vi "运维调试_总磷总氮.vi"() -> ()   [LabVIEW 2016, in "斯坦道总氮.lvlib"]
uses:
  <vilib>/Utility/miscctls.llb/LVPointTypeDef.ctl
  <vilib>/Plasmionique/MB Master/MB_Master/MB_Master.lvclass
  <vilib>/ptbypt/NI_PtbyPt.lvlib
panel:
  out "故障代码":u16
  out "告警代码":u16
  in  "产生故障":bool
  out "步骤":u16
  out "seconds since 1Jan1904 2":timestamp
  out "seconds since 1Jan1904":timestamp
  in  "周期设置":bool
  in  "流程操作":bool
  out "消解压力":sgl format="%#.2f kPa"
  out "权限等级":string
  out "总步数":i32
  out "滑动杆":dbl(slide) caption="测试进度" scale=0.0..100.0
  out "试剂余量显示":sgl[][](graph)
  in  "仪器校准":bool
  in  "参数查询":bool
  out "简易步骤名称":string
  in  "温度曲线":bool
  in  "试剂余量":bool
  in  "灯值调整":bool
  out "固件版本号":string
  out "模块版本号":string
  out "注射器温度":sgl format="%#.2f ℃"
  out "消解温度":sgl format="%#.2f ℃"
  out "ADC":sgl
  out "F3":sgl format="%#.6f"
  out "F2":sgl format="%#.6f"
  out "F1":sgl format="%#.6f"
  out "F0":sgl format="%#.6f"
  out "运行状态":T1 {"数据时间:" format="%<%y/%m/%d %H:%M:%S>T"; "仪器时间:" format="%<%y/%m/%d %H:%M:%S>T"}
  in  "单选按钮":T2=enum."总氮"
  in  "布尔":bool
  in  "外设固件":bool
  out "字符串 2":string
  in  "数组":string[](array[string])
  in  "返回":bool
  in  "参数设置":bool
  out "集成报警信息":string
  in  "停止":bool
  in  "手动启动":bool
  in  "调试":bool
  out "多列列表框":i32(listbox)
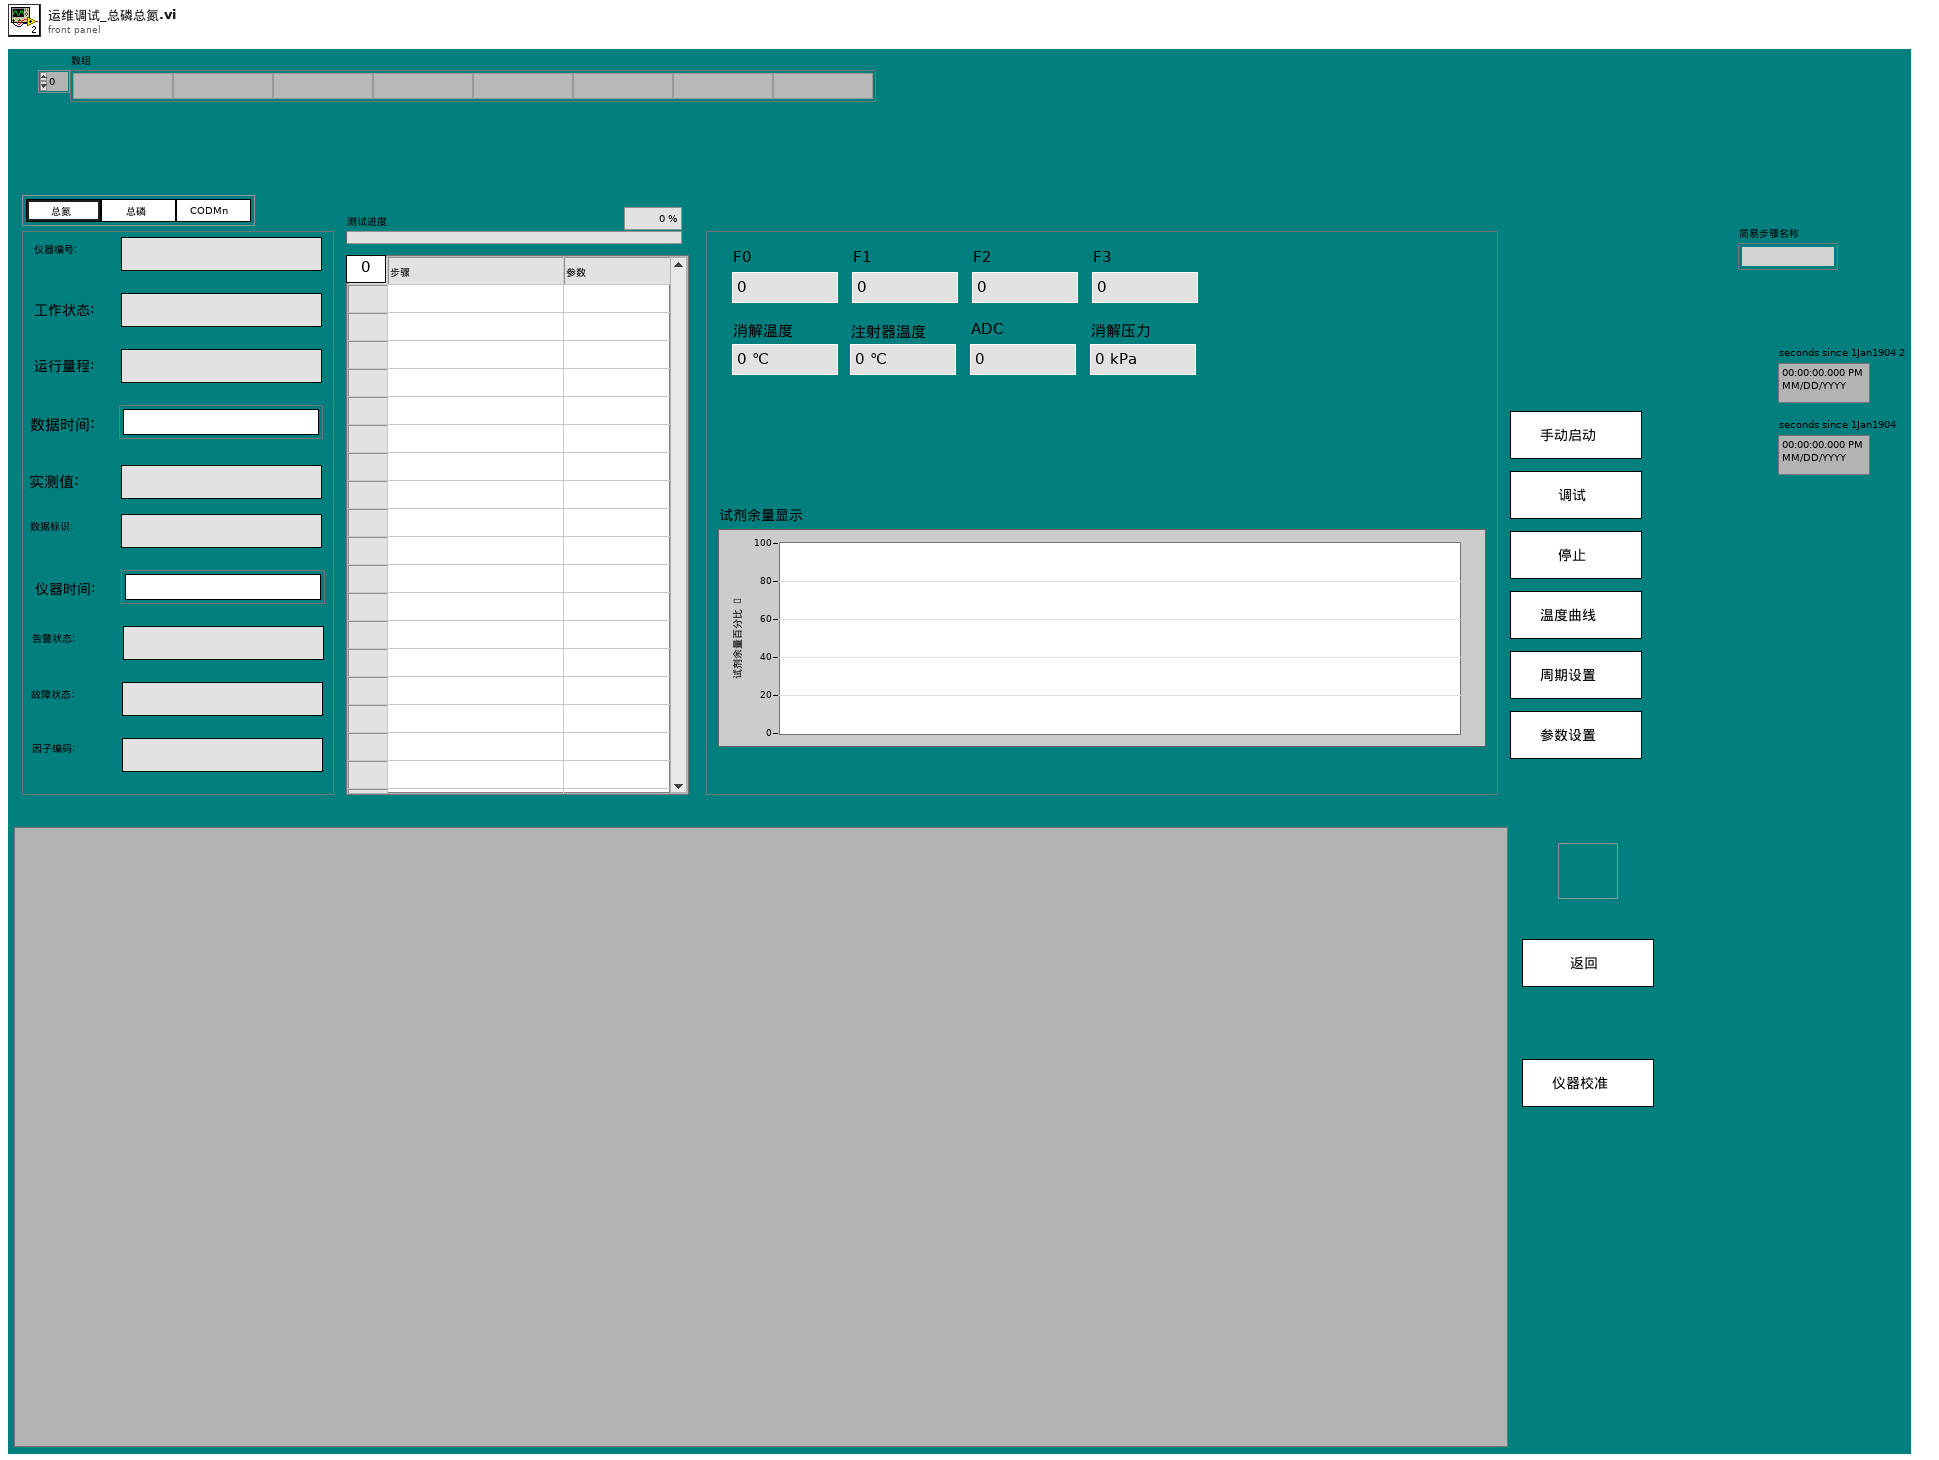
[diagram p1: front panel]
types:
  T1 = cluster{"仪器编号:":string, "工作状态:":string, "运行量程: ":string, "数据时间:":timestamp, "实测值:":string, "数据标识: ":string, "仪器时间:":timestamp, "告警状态: ":string, "故障状态:  ":string, "因子编码:":string}
  T2 = typedef "斯坦道总氮.lvlib/启动参数显示控件.ctl" = enum32{"COD", "氨氮", "总氮", "总磷", "磷酸盐", "硝氮", "亚硝氮", "硅酸盐", "硫化物", "氟化物", "CODMn"}
  T3 = typedef "报警信息字段定义.ctl" = cluster{"时间":timestamp, "参数":string, "元器件":string, "故障现象":string, "故障分析":string, "state":string, "code":string, "platform_alarm_code":string, "是否上报":string}
  T4 = cluster{"系统时间":timestamp, "工作状态":u16, "测量模式":enum16{"待机", "连续模式", "周期模式", "定点模式", "受控模式", "手动模式"}, "告警代码":u16, "故障代码":u16, "日志代码":u16, "软件版本":u16, "F0":sgl, "F1":sgl, "F2":sgl, "F3":sgl, "T":sgl, "H":sgl, "id":u16, "flowid":u16, "量程":u16, "总磷控温温度1":sgl, "营养盐控温温度2":sgl, "ADC":sgl, "结果值":sgl, "运行时间":u16, "步骤详情":string, "步骤流程":string}
  T5 = typedef "Alarm interface.lvlib/报警短信语音交互.ctl" = cluster{"参数":string, "元器件":string, "故障现象":string, "code":string, "platform_alarm_code":string, "solutionList":cluster{"reason":string, "solution":string}[], "是否上报":string}
  T6 = typedef "LVPointTypeDef.ctl" = cluster{"Horizontal":i16, "Vertical":i16}
  T7 = cluster{"Major":u16, "Minor":u16, "Fix":u16, "Build":u16}
  T8 = typedef "LVStringsAndValuesArrayTypeDef_U16.ctl" = cluster{"String":string, "Value":u16}[]
  T9 = cluster{"因子编码":u32, "单位":u16, "标样参考值":sgl, "水样数据时间":timestamp, "水样实测值":sgl, "水样数据标识":string, "标样数据时间":timestamp, "标样实测值":sgl, "标样数据标识":string, "空白数据时间":timestamp, "空白实测值":sgl, "空白数据标识":string, "零点核查数据时间":timestamp, "零点核查实测值":sgl, "零点核查数据标识":string, "跨度核查数据时间":timestamp, "跨度核查实测值":sgl, "跨度核查数据标识":string, "加标回收数据时间":timestamp, "加标回收实测值":sgl, "加标回收数据标识":string, "平行样数据时间":timestamp, "平行样实测值":sgl, "平行样数据标识":string, "F0":sgl, "F1":sgl, "F2":sgl, "F3":sgl, "F4":sgl, "F5":sgl, "F6":sgl, "F7":sgl, "温度":sgl, "湿度":sgl, "X值":sgl, "fidrange":u16, "X1值":sgl}[]
  T10 = typedef "SingleStepTestV3.lvlib/SingleStepTestV3.lvclass/仪器版本.ctl" = enum16{"V3.1版", "V4版", "V3版", "V4.2版"}
  T11 = cluster{"因子编码":u32, "单位":u16, "标样参考值":sgl, "水样数据时间":timestamp, "水样实测值":sgl, "水样数据标识":string, "标样数据时间":timestamp, "标样实测值":sgl, "标样数据标识":string, "空白数据时间":timestamp, "空白实测值":sgl, "空白数据标识":string, "零点核查数据时间":timestamp, "零点核查实测值":sgl, "零点核查数据标识":string, "跨度核查数据时间":timestamp, "跨度核查实测值":sgl, "跨度核查数据标识":string, "加标回收数据时间":timestamp, "加标回收实测值":sgl, "加标回收数据标识":string, "平行样数据时间":timestamp, "平行样实测值":sgl, "平行样数据标识":string, "F0":sgl, "F1":sgl, "F2":sgl, "F3":sgl, "F4":sgl, "F5":sgl, "F6":sgl, "F7":sgl, "温度":sgl, "湿度":sgl, "X值":sgl, "fidrange":u16, "X1值":sgl}
  T12 = typedef "TimingControl.lvlib/TimingControl.lvclass/国标控制命令.ctl" = enum16{"启动测量", "标样核查", "零点核查", "跨度核查", "空白测试", "平行样测试", "加标回收", "空白校准", "标样校准", "初始化（清洗）", "停止测试", "仪器重启", "校时", "模式设置", "测量间隔设置"}
  T13 = typedef "TimingControl.lvlib/TimingControl.lvclass/测量参数.ctl" = u16
  T14 = enum32{"Bad", "Idle", "Run top level", "Running"}
  T15 = cluster{"时间标识":timestamp, "设备":string, "日志信息":string, "流程参数":string}
  T16 = typedef "LVRowAndColumnUnsignedTypeDef.ctl" = cluster{"Row":u32, "Column":u32}
  T17 = typedef "操作日志字段定义.ctl" = cluster{"时间":timestamp, "参数":string, "日志信息":string, "流程参数":string}
  T18 = cluster{"站号":u16, "量程切换":enum32{"H", "L", "AUTO"}, "控制命令":enum16{"启动测量", "标样核查", "零点核查", "跨度核查", "空白测试", "平行样测试", "加标回收", "空白校准", "标样校准", "初始化（清洗）", "停止测试", "仪器重启", "校时", "模式设置", "测量间隔设置"}, "模式设置":enum16{"待机", "连续模式", "周期模式", "定点模式", "受控模式", "手动模式"}, "测量间隔":u16}
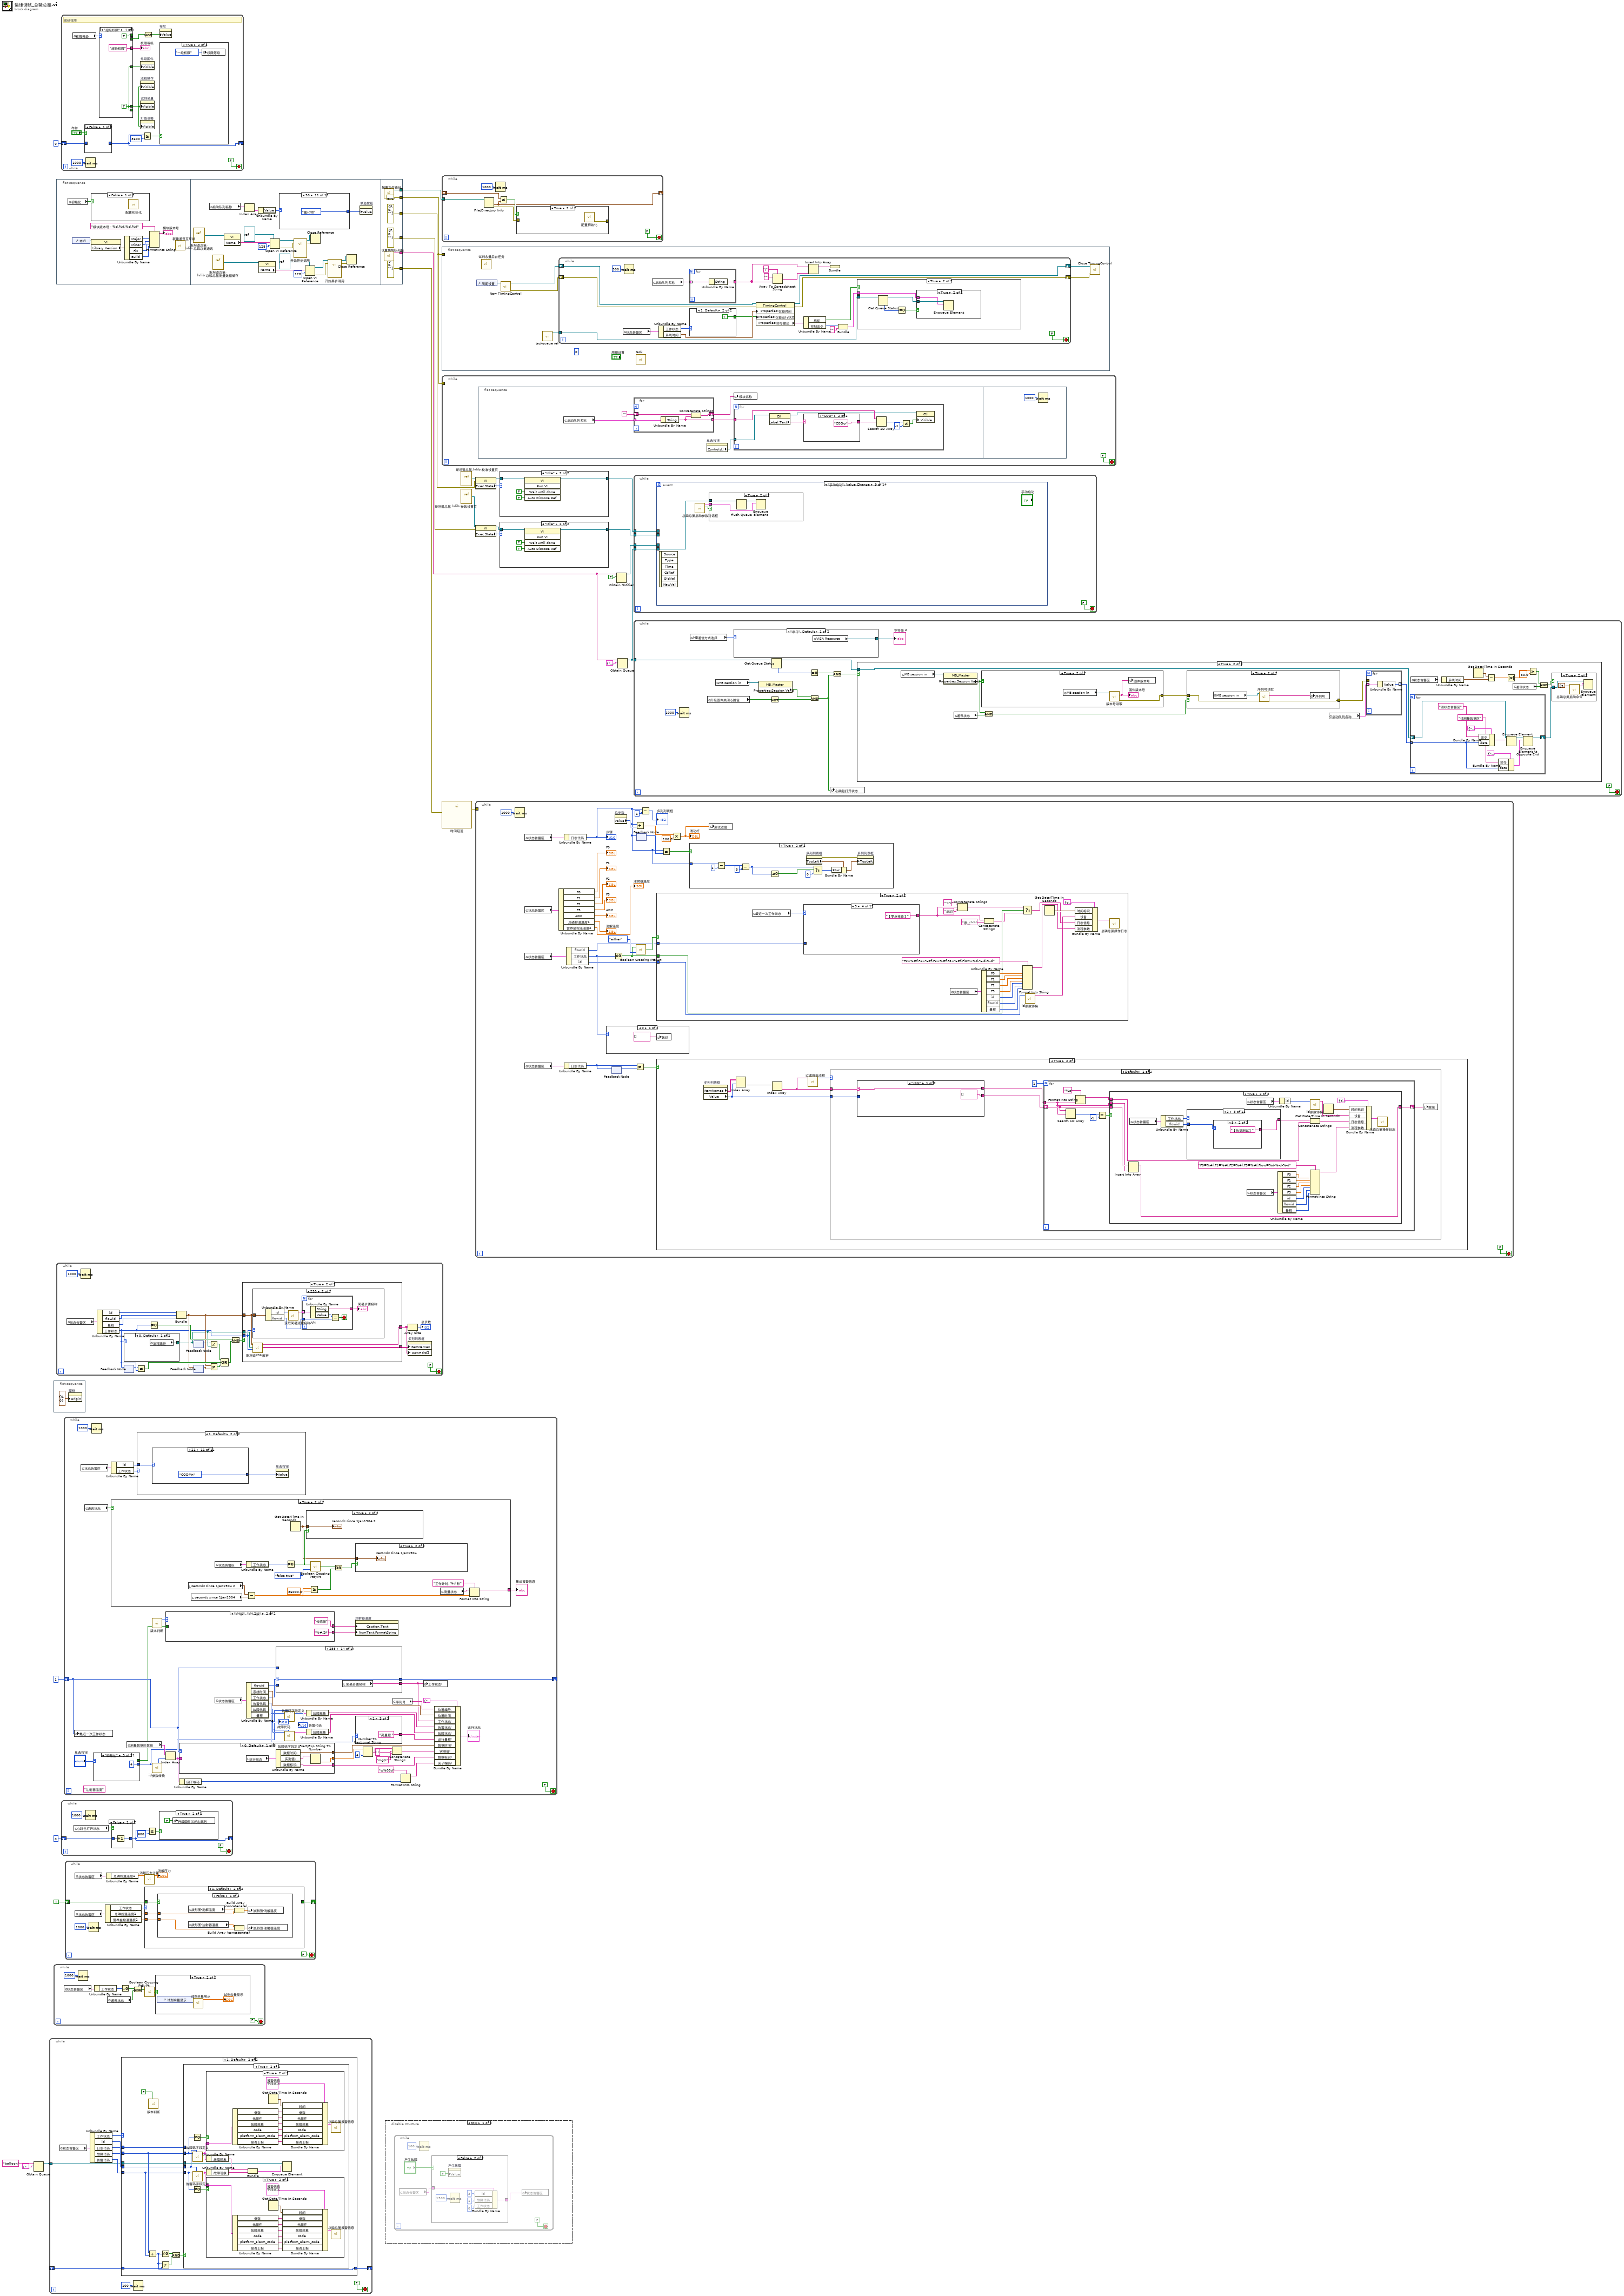
[diagram p0: block diagram]
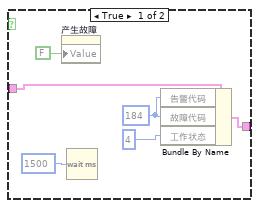
[diagram p2: hidden frame]
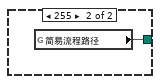
[diagram p8: hidden frame]
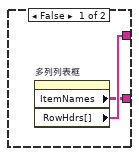
[diagram p9: hidden frame]
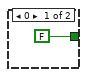
[diagram p13: hidden frame]
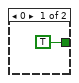
[diagram p20: hidden frame]
diagram:
  n1 = Obtain Queue(name (unnamed)="balloon" ("名称（未命名）"), element data type=cluster{"Title":string, "Body":string} {"Title"="", "Body"=""}) -> (queue out=w1:refnum<queue>)  [unwired: 3 in, 2 out]
  n2 = while {
    shift-right: [w29] -> _
    shift-left: _ -> [w31]
    tunnel: w1 -> [w28]
    stop <- FALSE stop-if-true
    n3 = global read "VAR总磷总氮全局变量.vi" "状态告警区"() -> (w27:T4)
    n4 = Unbundle By Name(w27) -> ("工作状态"=w36:u16, "id"=w35:u16, "日志代码"=w34:u16, "故障代码"=w33:u16, "告警代码"=w32:u16)
    n5 = case shown="1, Default" w36 {
      tunnel: w35 -> [_ w41]
      tunnel: w34 -> [_ w44]
      tunnel: w33 -> [_ w43]
      tunnel: w32 -> [_ w42]
      tunnel: w31 -> [w38 w47]
      tunnel: [w38 w45] -> w29
      tunnel: w28 -> [_ w40]
      frame 0 {
      }
      frame 1, Default {
        n6 = Add(x=w43, y=w42) -> (x+y=w45:u16)
        n7 = call "版本判断.vi"("Extern"=FALSE) -> ()  [unwired: 10 in, 1 out]
        n8 = Not Equal To 0?(x=w45) -> (x != 0?=w49:bool)
        n9 = Not Equal?(x=w45, y=w47) -> (x != y?=w48:bool)
        n10 = And(x=w49, y=w48) -> (x .and. y?=w46:bool)
        n11 = case shown="True" w46 {
          tunnel: w44 -> [_ _]
          tunnel: w43 -> [_ w54]
          tunnel: w42 -> [_ w51]
          tunnel: w41 -> [_ w50]
          tunnel: w40 -> [_ w58]
          frame False {
          }
          frame True {
            n12 = Not Equal To 0?(x=w54) -> (x != 0?=w56:bool)
            n13 = Not Equal To 0?(x=w51) -> (x != 0?=w55:bool)
            n14 = call "故障码字段定义.vi"("id"=w50, "故障代码"=w54) -> ("告警信息"=w53:T5)  [unwired: 9 in]
            n15 = call "告警码字段定义.vi"("id"=w50, "告警代码"=w51) -> ("告警信息"=w52:T5)  [unwired: 9 in]
            n16 = case shown="True" w56 {
              tunnel: w53 -> [_ w78]
              frame False {
              }
              frame True {
                n17 = Unbundle By Name(w78) -> ("参数"=w77:string, "元器件"=w76:string, "故障现象"=w75:string, "code"=w74:string, "platform_alarm_code"=w73:string, "是否上报"=w72:string)
                n18 = Get Date/Time In Seconds() -> (seconds since 1Jan1904=w79:timestamp)
                n19 = Bundle By Name(cluster=T3 {"时间"=timestamp(0 s since 1904-01-01), "参数"="", "元器件"="", "故障现象"="", "故障分析"="", "state"="", "code"="", "platform_alarm_code"="", "是否上报"=""} ("data in"), "时间"=w79, "参数"=w77, "元器件"=w76, "故障现象"=w75, "code"=w74, "platform_alarm_code"=w73, "是否上报"=w72) -> (w71:T3)
                n20 = call "总磷总氮报警信息.vi"("data in"=w71) -> ()  [unwired: 10 in, 1 out]
              }
            }
            n21 = Unbundle By Name(w53) -> ("故障现象"=w60:string)
            n22 = Unbundle By Name(w52) -> ("故障现象"=w59:string)
            n23 = case shown="True" w55 {
              tunnel: w52 -> [_ w62]
              frame False {
              }
              frame True {
                n24 = Unbundle By Name(w62) -> ("参数"=w65:string, "元器件"=w66:string, "故障现象"=w67:string, "code"=w68:string, "platform_alarm_code"=w69:string, "是否上报"=w70:string)
                n25 = Get Date/Time In Seconds() -> (seconds since 1Jan1904=w64:timestamp)
                n26 = Bundle By Name(cluster=T3 {"时间"=timestamp(0 s since 1904-01-01), "参数"="", "元器件"="", "故障现象"="", "故障分析"="", "state"="", "code"="", "platform_alarm_code"="", "是否上报"=""} ("data in"), "时间"=w64, "参数"=w65, "元器件"=w66, "故障现象"=w67, "code"=w68, "platform_alarm_code"=w69, "是否上报"=w70) -> (w61:T3)
                n27 = call "总磷总氮报警信息.vi"("data in"=w61) -> ()  [unwired: 10 in, 1 out]
              }
            }
            n28 = Bundle("故障现象"=w60, "故障现象"=w59) -> (w57:cluster{"故障现象":string, "故障现象":string})  [unwired: 1 in]
            n29 = Enqueue Element(queue=w58, element=w57) -> ()  [unwired: 2 in, 3 out]
          }
        }
      }
    }
    n30 = Wait (ms)(milliseconds to wait=u32 100 ("等待时间（毫秒）")) -> ()  [unwired: 1 out]
  }
  n31 = flat-sequence {
    frame #0 {
      n32 = property on="窗格" class="Pane"("Origin"=T6 {"Horizontal"=0, "Vertical"=0} ("原点")) -> ()  [unwired: 2 in, 2 out]
    }
  }
  n33 = while {
    stop <- FALSE stop-if-true
    n34 = global read "VAR总磷总氮全局变量.vi" "状态告警区"() -> (w86:T4)
    n35 = Wait (ms)(milliseconds to wait=u32 1000 ("等待时间（毫秒）")) -> ()  [unwired: 1 out]
    n36 = Unbundle By Name(w86) -> ("工作状态"=w84:u16)
    n37 = global read "VAR总磷总氮全局变量.vi" "通讯状态"() -> (w87:bool)
    n38 = Equal To 0?(x=w84) -> (x = 0?=w83:bool)
    n39 = And(x=w83, y=w87) -> (x .and. y?=w85:bool)
    n40 = call <vilib>:"Boolean Crossing PtByPt.vi"("input"=w85) -> ("crossing"=w82:bool)  [unwired: 2 in]
    n41 = case shown="True" w82 {
      frame False {
      }
      frame True {
        n42 = control-ref of="试剂余量显示"() -> (w90:refnum<vi>)
        n43 = call "试剂余量展示.vi"("波形图 2"=w90) -> ("波形图"=→"试剂余量显示":sgl[][])  [unwired: 10 in]
      }
    }
  }
  n44 = flat-sequence {
    tunnel: [w138] -> w20
    tunnel: [errorcluster {"status"=FALSE, "code"=0, "source"=""} ("错误输入（无错误）")] -> w11
    tunnel: [errorcluster {"status"=FALSE, "code"=0, "source"=""} ("错误输入（无错误）")] -> w10
    tunnel: [w135] -> w8
    tunnel: [errorcluster {"status"=FALSE, "code"=0, "source"=""} ("error out")] -> w7
    tunnel: [errorcluster {"status"=FALSE, "code"=0, "source"=""} ("错误输入（无错误）")] -> w6
    frame #0 {
      n45 = global read "VAR总磷总氮全局变量.vi" "初始化"() -> (w92:bool)
      n46 = control-ref of="本VI"() -> (w100:refnum<vi>)
      n47 = case shown="False" w92 {
        frame False {
          n48 = call "配置初始化.vi"() -> ()  [unwired: 11 in, 1 out]
        }
        frame True {
        }
      }
      n49 = property class="VI"(reference=w100) -> ("Library.Version"=w99:T7)  [unwired: 1 in, 2 out]
      n50 = Unbundle By Name(w99) -> ("Major"=w97:u16, "Minor"=w96:u16, "Fix"=w95:u16, "Build"=w94:u16)
      n51 = Format Into String(format string="模块版本号：%d.%d.%d.%d" ("格式字符串"), w97, w96, w95, w94) -> (resulting string=→"模块版本号":string)  [unwired: 2 in, 1 out]
      n52 = call "新建通讯互斥锁.vi"() -> ()  [unwired: 11 in, 1 out]
    }
    frame #1 {
      n53 = vi-ref "斯坦道总氮.lvlib:总磷总氮通讯.vi"() -> (w105:refnum<vi>)
      n54 = global read "model config var.vi" "启动队列名称"() -> (w103:cluster{"String":string, "Value":u16}[])
      n55 = vi-ref "斯坦道总氮.lvlib:总磷总氮测量数据储存.vi"() -> (w113:refnum<vi>)
      n56 = property class="VI"(reference=w105) -> ("Name"=w106:string)  [unwired: 1 in, 2 out]
      n57 = Index Array(array=w103) -> (element=w102:cluster{"String":string, "Value":u16})  [unwired: 1 in]
      n58 = Unbundle By Name(w102) -> ("Value"=w101:u16)
      n59 = property class="VI"(reference=w113) -> ("Name"=w120:string)  [unwired: 1 in, 2 out]
      n60 = Open VI Reference(type specifier VI Refnum (for type only)=refnum<vi> refnum, vi path=w106, options=128 ("选项")) -> (vi reference=w108:refnum<vi>, error out=w110:errorcluster)  [unwired: 3 in]
      n61 = case shown="50" w101 {
        tunnel: [w121 启动参数显示控件."总磷" ("单选按钮") 启动参数显示控件."总氮" ("单选按钮") 启动参数显示控件."COD" ("单选按钮") 启动参数显示控件."氨氮" ("单选按钮") 启动参数显示控件."磷酸盐" ("单选按钮") 启动参数显示控件."硝氮" ("单选按钮") 启动参数显示控件."亚硝氮" ("单选按钮") 启动参数显示控件."硅酸盐" ("单选按钮") 启动参数显示控件."硫化物" ("单选按钮") 启动参数显示控件."氟化物" ("单选按钮") 启动参数显示控件."CODMn" ("单选按钮")] -> w104
        frame 0, Default {
          n62 = property on="单选按钮" class="RadioBtnsControl (strict)"() -> ("Value"=w121:T2)  [unwired: 2 in, 2 out]
        }
        frame 1 {
        }
        frame 2 {
        }
        frame 22 {
        }
        frame 3 {
        }
        frame 4 {
        }
        frame 5 {
        }
        frame 6 {
        }
        frame 7 {
        }
        frame 8 {
        }
        frame 50 {
        }
        frame 21 {
        }
      }
      n63 = call-by-ref "开始异步调用"(reference=w108, error in=w110) -> (reference out=w112:refnum<vi>, error out=w111:errorcluster)  [unwired: 12 in]
      n64 = Open VI Reference(type specifier VI Refnum (for type only)=refnum<vi> refnum, vi path=w120, options=128 ("选项")) -> (vi reference=w118:refnum<vi>, error out=w116:errorcluster)  [unwired: 3 in]
      n65 = Close Reference(reference=w112, error in (no error)=w111) -> ()  [unwired: 1 out]
      n66 = call-by-ref "开始异步调用"(reference=w118, error in=w116) -> (reference out=w114:refnum<vi>, error out=w115:errorcluster)  [unwired: 12 in]
      n67 = Close Reference(reference=w114, error in (no error)=w115) -> ()  [unwired: 1 out]
      n68 = property on="单选按钮" class="RadioBtnsControl (strict)"("Value"=w104) -> ()  [unwired: 2 in, 2 out]
    }
    frame #2 {
      n69 = call "配置文件路径.vi"() -> ("appended path"=w135:path)  [unwired: 11 in]
      n70 = call "设置模块队列名.vi"() -> ("Msg"=w138:string)  [unwired: 5 in]
    }
  }
  n71 = while {
    stop <- FALSE stop-if-true
    n72 = global read "VAR总磷总氮全局变量.vi" "状态告警区"() -> (w150:T4)
    n73 = Wait (ms)(milliseconds to wait=u32 1000 ("等待时间（毫秒）")) -> ()  [unwired: 1 out]
    n74 = Unbundle By Name(w150) -> ("id"=w149:u16, "flowid"=w148:u16, "量程"=w147:u16, "工作状态"=w140:u16)
    n75 = case shown="0, Default" w140 {
      tunnel: [w160 w161] -> w142
      frame 0, Default {
        n76 = global read "总磷总氮断电保存全局变量.vi" "流程路径"() -> (w160:path)
      }
      frame 255 {
        n77 = global read "总磷总氮断电保存全局变量.vi" "简易流程路径"() -> (w161:path)
      }
    }
    n78 = feedback #1() -> (w139:u16)  [unwired: 1 in]
    n79 = feedback-in #1(w140) -> ()
    n80 = Not Equal?(x=w139, y=w140) -> (x != y?=w156:bool)
    n81 = Not Equal To 0?(x=w140) -> (x != 0?=w151:bool)
    n82 = Bundle("id"=w149, "flowid"=w148, "量程"=w147) -> (w144:cluster{"id":u16, "flowid":u16, "量程":u16})  [unwired: 1 in]
    n83 = feedback #2() -> (w141:path)  [unwired: 1 in]
    n84 = feedback-in #2(w142) -> ()
    n85 = feedback-in #3(w144) -> ()
    n86 = feedback #3() -> (w145:cluster{"id":u16, "flowid":u16, "量程":u16})  [unwired: 1 in]
    n87 = Not Equal?(x=w141, y=w142) -> (x != y?=w155:bool)
    n88 = Not Equal?(x=w144, y=w145) -> (x != y?=w143:bool)
    n89 = Compound Arithmetic op=OR ("复合运算")(w155, w156, w143) -> (w157:bool)
    n90 = And(x=w151, y=w157) -> (x .and. y?=w152:bool)
    n91 = case shown="True" w152 {
      tunnel: [w163 w166] -> w154
      tunnel: [w162 w167] -> w158
      tunnel: w144 -> [_ w165]
      tunnel: w142 -> [_ w168]
      tunnel: w140 -> [_ w164]
      frame False {
        n92 = property on="多列列表框" class="MCListbox (strict)"() -> ("ItemNames"=w162:string[][], "RowHdrs[]"=w163:string[])  [unwired: 2 in, 2 out]
      }
      frame True {
        n93 = case shown="255" w164 {
          tunnel: w165 -> [_ w173]
          frame 0, Default {
          }
          frame 255 {
            n94 = Unbundle By Name(w173) -> ("id"=w172:u16, "flowid"=w170:u16)
            n95 = call "获取简易流程名称API.vi"("参数下拉列表"=w172) -> ("字符串与值[]"=w171:T8)  [unwired: 9 in, 1 out]
            n96 = for {
              tunnel: w171 -> [w178] mode=indexing
              tunnel: w170 -> [w176]
              tunnel: [w175] -> w169
              stop <- w174 stop-if-true
              n97 = Unbundle By Name(w178) -> ("String"=w175:string, "Value"=w177:u16)
              n98 = Equal?(x=w177, y=w176) -> (x = y?=w174:bool)
            }
            "简易步骤名称" <- w169
          }
        }
        n99 = call "斯坦道XML解析.vi"("工作状态"=w164, "添加的路径"=w168, "参数簇"=w165) -> ("步骤名"=w167:string[][], "索引"=w166:string[])  [unwired: 6 in, 1 out]
      }
    }
    n100 = Array Size(array=w154) -> (size(s)=→"总步数":i32)
    n101 = property on="多列列表框" class="MCListbox (strict)"("ItemNames"=w158, "RowHdrs[]"=w154) -> ()  [unwired: 2 in, 2 out]
  }
  n102 = while {
    shift-right: [w188] -> _
    shift-left: u32 0 ("y") -> [w190]
    stop <- FALSE stop-if-true
    # "密码权限"
    n103 = global read "VAR总磷总氮全局变量.vi" "权限等级"() -> (w185:enum16{"一级权限", "二级权限", "三级权限", "超级权限"})
    n104 = case shown="False" "布尔" {
      tunnel: w190 -> [_ w203]
      tunnel: [_ w202] -> w188
      frame False {
      }
      frame True {
        n105 = Increment(x=w203) -> (x+1=w202:u32)
      }
    }
    n106 = Wait (ms)(milliseconds to wait=u32 1000 ("等待时间（毫秒）")) -> ()  [unwired: 1 out]
    n107 = case shown="\"超级权限\"" w185 {
      tunnel: [_ w195 w197 w200] -> w179
      tunnel: [_ _ w197 w200] -> _
      tunnel: [_ w195 w197 w200] -> w184
      tunnel: [_ _ _ TRUE] -> _
      tunnel: [TRUE _ _ _] -> w182
      tunnel: ["一级权限" "二级权限" "三级权限" "超级权限"] -> w180
      frame "一级权限", Default {
      }
      frame "二级权限" {
        w195 = TRUE
      }
      frame "三级权限" {
        w197 = TRUE
      }
      frame "超级权限" {
        w200 = TRUE
      }
    }
    "权限等级" <- w180
    n108 = property on="外设固件" class="Bool"("Visible"=w184) -> ()  [unwired: 2 in, 2 out]
    n109 = property on="流程操作" class="Bool"("Visible"=w179) -> ()  [unwired: 2 in, 2 out]
    n110 = property on="试剂余量" class="Bool"("Visible"=w179) -> ()  [unwired: 2 in, 2 out]
    n111 = property on="灯值调整" class="Bool"("Visible"=w179) -> ()  [unwired: 2 in, 2 out]
    n112 = Greater Or Equal?(x=w188, y=u32 3600) -> (x >= y?=w186:bool)
    n113 = Not(x=w182) -> (.not. x?=w181:bool)
    n114 = property on="布尔" class="Bool (strict)"("Value"=w181) -> ()  [unwired: 2 in, 2 out]
    n115 = case shown="True" w186 {
      frame False {
      }
      frame True {
        n116 = global write "VAR总磷总氮全局变量.vi" "权限等级"(enum16{"一级权限", "二级权限", "三级权限", "超级权限"}."一级权限" ("权限等级")) -> ()
      }
    }
  }
  n117 = while {
    shift-right: [w208] -> _
    shift-left: 0 -> [w209]
    stop <- FALSE stop-if-true
    n118 = global read "VAR总磷总氮全局变量.vi" "心跳包打开状态"() -> (w204:bool)
    n119 = Wait (ms)(milliseconds to wait=u32 1000 ("等待时间（毫秒）")) -> ()  [unwired: 1 out]
    n120 = case shown="False" w204 {
      tunnel: w209 -> [w213 _]
      tunnel: [w212 _] -> w208
      frame False {
        n121 = Increment(x=w213) -> (x+1=w212:i32)
      }
      frame True {
      }
    }
    n122 = Greater Or Equal?(x=w208, y=600) -> (x >= y?=w206:bool)
    n123 = case shown="True" w206 {
      frame False {
      }
      frame True {
        n124 = global write "VAR总磷总氮全局变量.vi" "升级固件关闭心跳包"(FALSE ("关闭心跳包")) -> ()
      }
    }
  }
  n125 = while {
    shift-right: [w225] -> _
    shift-left: u16 1 ("工作状态") -> [w223]
    stop <- FALSE stop-if-true
    (unwired) "注射器温度"
    n126 = global write "VAR总磷总氮全局变量.vi" "最近一次工作状态"(w223) -> ()
    n127 = global read "VAR总磷总氮全局变量.vi" "状态告警区"() -> (w245:T4)
    n128 = global read "VAR总磷总氮全局变量.vi" "通讯状态"() -> (w256:bool)
    n129 = Wait (ms)(milliseconds to wait=u32 1000 ("等待时间（毫秒）")) -> ()  [unwired: 1 out]
    n130 = case shown="\"磷酸盐\"" "单选按钮" {
      tunnel: [22 3 2 1 4 5 6 7 8 50 21] -> w214
      tunnel: [_ TRUE _ _ _ _ _ _ _ _ _] -> w217
      frame "COD", Default {
      }
      frame "氨氮" {
      }
      frame "总氮" {
      }
      frame "总磷" {
      }
      frame "磷酸盐" {
      }
      frame "硝氮" {
      }
      frame "亚硝氮" {
      }
      frame "硅酸盐" {
      }
      frame "硫化物" {
      }
      frame "氟化物" {
      }
      frame "CODMn" {
      }
    }
    n131 = Unbundle By Name(w245) -> ("id"=w244:u16, "工作状态"=w240:u16)
    n132 = case shown="True" w256 {
      tunnel: ["通讯异常" ("集成报警信息") w375] -> w255
      frame False {
      }
      frame True {
        n133 = local read "seconds since 1Jan1904 2"() -> (w367:timestamp)
        n134 = local read "seconds since 1Jan1904"() -> (w370:timestamp)
        n135 = global read "VAR总磷总氮全局变量.vi" "状态告警区"() -> (w377:T4)
        n136 = Unbundle By Name(w377) -> ("工作状态"=w373:u16)
        n137 = Subtract(x=w367, y=w370) -> (x-y=w366:dbl)
        n138 = Not Equal To 0?(x=w373) -> (x != 0?=w369:bool)
        n139 = Get Date/Time In Seconds() -> (seconds since 1Jan1904=w368:timestamp)
        n140 = case shown="True" w369 {
          tunnel: w368 -> [_ w378]
          frame False {
          }
          frame True {
            "seconds since 1Jan1904 2" <- w378
          }
        }
        n141 = Greater Or Equal?(x=w366, y=36000.0) -> (x >= y?=w363:bool)
        n142 = call <vilib>:"Boolean Crossing PtByPt.vi"("direction"=enum16{"either", "false-true", "true-false"}."false-true", "input"=w369) -> ("crossing"=w371:bool)  [unwired: 1 in]
        n143 = Or(x=w371, y=w363) -> (x .or. y?=w364:bool)
        n144 = case shown="True" w364 {
          tunnel: w368 -> [_ w379]
          frame False {
          }
          frame True {
            "seconds since 1Jan1904" <- w379
          }
        }
        n145 = global read "VAR总磷总氮全局变量.vi" "测量状态"() -> (w374:string)
        n146 = Format Into String(format string="工作计时: %d 秒" ("格式字符串"), initial string=w374, w366) -> (resulting string=w375:string)  [unwired: 1 in, 1 out]
      }
    }
    "集成报警信息" <- w255
    n147 = global read "VAR总磷总氮全局变量.vi" "测量数据区数组"() -> (w229:T9)
    n148 = case shown="1, Default" w240 {
      tunnel: w244 -> [_ w312]
      frame 0 {
      }
      frame 1, Default {
        n149 = case shown="21" w312 {
          tunnel: [w313 启动参数显示控件."总磷" ("单选按钮") 启动参数显示控件."总氮" ("单选按钮") 启动参数显示控件."COD" ("单选按钮") 启动参数显示控件."氨氮" ("单选按钮") 启动参数显示控件."磷酸盐" ("单选按钮") 启动参数显示控件."硝氮" ("单选按钮") 启动参数显示控件."亚硝氮" ("单选按钮") 启动参数显示控件."硅酸盐" ("单选按钮") 启动参数显示控件."硫化物" ("单选按钮") 启动参数显示控件."CODMn" ("单选按钮") 启动参数显示控件."氟化物" ("单选按钮")] -> w311
          frame 0, Default {
            n150 = property on="单选按钮" class="RadioBtnsControl (strict)"() -> ("Value"=w313:T2)  [unwired: 2 in, 2 out]
          }
          frame 1 {
          }
          frame 2 {
          }
          frame 22 {
          }
          frame 3 {
          }
          frame 4 {
          }
          frame 5 {
          }
          frame 6 {
          }
          frame 7 {
          }
          frame 8 {
          }
          frame 21 {
          }
          frame 50 {
          }
        }
        n151 = property on="单选按钮" class="RadioBtnsControl (strict)"("Value"=w311) -> ()  [unwired: 2 in, 2 out]
      }
    }
    n152 = call "版本判断.vi"() -> ("仪器版本"=w219:T10)  [unwired: 11 in]
    n153 = call "id参数转换.vi"("id"=w214) -> ("数组资源索引"=w226:i32)  [unwired: 9 in, 1 out]
    n154 = case shown="\"V4版\", \"V4.2版\"" w219 {
      tunnel: [w259 "传感器" ("标题.文本")] -> w216
      tunnel: ["%#.2f ℃" ("数值文本.格式字符串") "%#.2f " ("数值文本.格式字符串")] -> w218
      tunnel: w217 -> [w262 _]
      frame "V3.1版", Default {
        n155 = Select(t="显色温度", s=w262, f="注射器温度" ("标题.文本")) -> (s? t:f=w259:string)
      }
      frame "V4版", "V4.2版" {
      }
    }
    n156 = Index Array(array=w229, index=w226) -> (element=w228:T11)
    n157 = case shown="0, Default" w223 {
      tunnel: [w280 w286 w290 w294 w298 w302 w306 w310] -> w239
      tunnel: [w278 w285 w289 w293 w296 w301 w305 w309] -> w234
      tunnel: [w281 w284 w288 w292 w295 w300 w304 w308] -> w232
      tunnel: w228 -> [_ w283 w287 w291 w297 w299 w303 w307]
      frame 0, Default {
        n158 = local read "运行状态"() -> (w282:T1)
        n159 = Unbundle By Name(w282) -> ("数据时间:"=w280:timestamp, "实测值:"=w279:string, "数据标识:"=w281:string)
        n160 = Fract/Exp String To Number(string=w279) -> (number=w278:dbl)  [unwired: 3 in, 1 out]
      }
      frame 1 {
        n161 = Unbundle By Name(w283) -> ("水样数据时间"=w286:timestamp, "水样实测值"=w285:sgl, "水样数据标识"=w284:string)
      }
      frame 2, 9 {
        n162 = Unbundle By Name(w287) -> ("标样数据时间"=w290:timestamp, "标样实测值"=w289:sgl, "标样数据标识"=w288:string)
      }
      frame 3 {
        n163 = Unbundle By Name(w291) -> ("零点核查数据时间"=w294:timestamp, "零点核查实测值"=w293:sgl, "零点核查数据标识"=w292:string)
      }
      frame 4 {
        n164 = Unbundle By Name(w297) -> ("跨度核查数据时间"=w298:timestamp, "跨度核查实测值"=w296:sgl, "跨度核查数据标识"=w295:string)
      }
      frame 7 {
        n165 = Unbundle By Name(w299) -> ("加标回收数据时间"=w302:timestamp, "加标回收实测值"=w301:sgl, "加标回收数据标识"=w300:string)
      }
      frame 5, 8 {
        n166 = Unbundle By Name(w303) -> ("空白数据时间"=w306:timestamp, "空白实测值"=w305:sgl, "空白数据标识"=w304:string)
      }
      frame 6 {
        n167 = Unbundle By Name(w307) -> ("平行样数据时间"=w310:timestamp, "平行样实测值"=w309:sgl, "平行样数据标识"=w308:string)
      }
    }
    n168 = Unbundle By Name(w228) -> ("因子编码"=w230:u32)
    n169 = global read "VAR总磷总氮全局变量.vi" "状态告警区"() -> (w254:T4)
    n170 = Unbundle By Name(w254) -> ("flowid"=w222:u16, "系统时间"=w250:timestamp, "工作状态"=w249:u16, "告警代码"=w243:u16, "故障代码"=w242:u16, "量程"=w248:u16)
    "告警代码" <- w243
    "故障代码" <- w242
    n171 = case shown="255" w249 {
      selector: w249 -> [w329 _ w335 w339 w342 w344 w346 w348 w350 w352 w354 w356 w358 w361]
      tunnel: [w330 "空闲" ("工作状态") "水样测量" ("工作状态") w338 "零点核查" ("工作状态") "跨度核查" ("工作状态") "空白测试" ("工作状态") "平行样测试" ("工作状态") "加标回收" ("工作状态") "空白校准" ("工作状态") "标样校准" ("工作状态") "初始化" ("工作状态") "单步调试" ("工作状态") w360] -> w224
      tunnel: [w328 w333 w335 w339 w342 w344 w346 w348 w350 w352 w354 w356 w358 w361] -> w225
      tunnel: w223 -> [w328 w333 _ _ _ _ _ _ _ _ _ _ _ _]
      tunnel: w222 -> [_ _ _ w337 _ _ _ _ _ _ _ _ _ _]
      frame Default {
        n172 = Format Into String(format string="%d" ("格式字符串"), initial string="未知" ("工作状态"), w329) -> (resulting string=w330:string)  [unwired: 1 in, 1 out]
      }
      frame 0 {
      }
      frame 1 {
      }
      frame 2 {
        n173 = case shown="5" w337 {
          tunnel: ["标样核查" ("工作状态") "快捷测试" ("工作状态")] -> w338
          frame 0, Default {
          }
          frame 5 {
          }
        }
      }
      frame 3 {
      }
      frame 4 {
      }
      frame 5 {
      }
      frame 6 {
      }
      frame 7 {
      }
      frame 8 {
      }
      frame 9 {
      }
      frame 10 {
      }
      frame 254 {
      }
      frame 255 {
        n174 = local read "简易步骤名称"() -> (w360:string)
      }
    }
    n175 = call "告警码字段定义.vi"("id"=w214, "告警代码"=w243) -> ("告警信息"=w221:T5)  [unwired: 9 in]
    n176 = call "故障码字段定义.vi"("id"=w214, "故障代码"=w242) -> ("告警信息"=w241:T5)  [unwired: 9 in]
    n177 = Unbundle By Name(w221) -> ("故障现象"=w220:string)
    n178 = Unbundle By Name(w241) -> ("故障现象"=w215:string)
    n179 = property on="注射器温度" class="DigNum (strict)"("Caption.Text"=w216, "NumText.FormatString"=w218) -> ()  [unwired: 2 in, 2 out]
    n180 = case shown="1" w248 {
      tunnel: ["" ("字符串") "低量程 " ("字符串") "高量程 " ("字符串")] -> w247
      frame Default {
      }
      frame 0 {
      }
      frame 1 {
      }
    }
    n181 = Number To Fractional String(number=w234, precision (6)=i16 4 ("精度(6)")) -> (F-format string=w236:string)  [unwired: 2 in]
    n182 = Concatenate Strings(w236, " " ("字符串"), "mg/L" ("字符串")) -> (w233:string)
    n183 = global read "VAR总磷总氮全局变量.vi" "序列号"() -> (w251:string)
    n184 = Format Into String(format string="w%05d" ("格式字符串"), w230) -> (resulting string=w246:string)  [unwired: 2 in, 1 out]
    n185 = global write "VAR总磷总氮全局变量.vi" "工作状态:"(w224) -> ()
    n186 = Bundle By Name(cluster=T1 {"仪器编号:"="", "工作状态:"="", "运行量程: "="", "数据时间:"=timestamp(0 s since 1904-01-01), "实测值:"="", "数据标识: "="", "仪器时间:"=timestamp(0 s since 1904-01-01), "告警状态: "="", "故障状态:  "="", "因子编码:"=""} ("运行状态"), "仪器编号:"=w251, "仪器时间:"=w250, "工作状态:"=w224, "告警状态:"=w220, "故障状态:"=w215, "运行量程:"=w247, "数据时间:"=w239, "实测值:"=w233, "数据标识:"=w232, "因子编码:"=w246) -> (→"运行状态":T1)
  }
  n187 = while {
    shift-right: [w381] -> _
    shift-left: TRUE -> [w382]
    stop <- FALSE stop-if-true
    n188 = global read "VAR总磷总氮全局变量.vi" "状态告警区"() -> (w385:T4)
    n189 = global read "VAR总磷总氮全局变量.vi" "状态告警区"() -> (w388:T4)
    n190 = Wait (ms)(milliseconds to wait=u32 1000 ("等待时间（毫秒）")) -> ()  [unwired: 1 out]
    n191 = Unbundle By Name(w388) -> ("工作状态"=w383:u16, "总磷控温温度1"=w387:sgl, "营养盐控温温度2"=w386:sgl)
    n192 = Unbundle By Name(w385) -> ("总磷控温温度1"=w384:sgl)
    n193 = call "消解压力计算.vi"("当前消解温度"=w384) -> ("消解压力"=→"消解压力":dbl)  [unwired: 10 in]
    n194 = case shown="1, Default" w383 {
      tunnel: w387 -> [_ w394]
      tunnel: w386 -> [_ w393]
      tunnel: w382 -> [_ w392]
      tunnel: [TRUE _] -> w381
      frame 0 {
      }
      frame 1, Default {
        n195 = case shown="False" w392 {
          tunnel: w394 -> [w400 _]
          tunnel: w393 -> [w399 _]
          frame False {
            n196 = global read "VAR总磷总氮全局变量.vi" "波形图-消解温度"() -> (w398:sgl[])
            n197 = global read "VAR总磷总氮全局变量.vi" "波形图-注射器温度"() -> (w397:sgl[])
            n198 = Build Array (concatenate)(w398, w400) -> (w396:sgl[])
            n199 = Build Array (concatenate)(w397, w399) -> (w395:sgl[])
            n200 = global write "VAR总磷总氮全局变量.vi" "波形图-消解温度"(w396) -> ()
            n201 = global write "VAR总磷总氮全局变量.vi" "波形图-注射器温度"(w395) -> ()
          }
          frame True {
            w401 = dbl[] [] ("波形图-消解温度")
            n202 = global write "VAR总磷总氮全局变量.vi" "波形图-消解温度"(w401) -> ()
            n203 = global write "VAR总磷总氮全局变量.vi" "波形图-注射器温度"(w401) -> ()
          }
        }
      }
    }
  }
  n204 = disable-structure shown="禁用" {
    frame Disabled {
      n205 = while {
        stop <- FALSE stop-if-true
        n206 = global read "VAR总磷总氮全局变量.vi" "状态告警区"() -> (w403:T4)
        n207 = Wait (ms)(milliseconds to wait=u32 100 ("等待时间（毫秒）")) -> ()  [unwired: 1 out]
        n208 = case shown="False" "产生故障" {
          tunnel: [w409 w415] -> w402
          tunnel: w403 -> [w408 w413]
          frame True {
            w407 = u16 184 ("故障代码")
            n209 = property on="产生故障" class="Bool (strict)"("Value"=FALSE ("产生故障")) -> ()  [unwired: 2 in, 2 out]
            n210 = Wait (ms)(milliseconds to wait=u32 1500 ("等待时间（毫秒）")) -> ()  [unwired: 1 out]
            n211 = Bundle By Name(cluster=w408, "告警代码"=w407, "故障代码"=w407, "工作状态"=u16 4) -> (w409:T4)
          }
          frame False {
            n212 = property on="产生故障" class="Bool (strict)"("Value"=FALSE ("产生故障")) -> ()  [unwired: 2 in, 2 out]
            n213 = Wait (ms)(milliseconds to wait=u32 1500 ("等待时间（毫秒）")) -> ()  [unwired: 1 out]
            n214 = Bundle By Name(cluster=w413, "id"=u16 3, "故障代码"=u16 1, "工作状态"=u16 0) -> (w415:T4)
          }
        }
        n215 = global write "VAR总磷总氮全局变量.vi" "状态告警区"(w402) -> ()
      }
    }
    frame Enabled {
    }
  }
  n216 = while {
    shift-right: [w420] -> _
    shift-left: _ -> [w425]
    tunnel: w8 -> [w423]
    stop <- FALSE stop-if-true
    n217 = File/Directory Info(path=w423) -> (last mod=w420:timestamp, error out=w421:errorcluster)  [unwired: 1 in, 5 out]
    n218 = Wait (ms)(milliseconds to wait=u32 1000 ("等待时间（毫秒）")) -> ()  [unwired: 1 out]
    n219 = Not Equal?(x=w425, y=w420) -> (x != y?=w424:bool)
    n220 = case shown="True" w424 {
      tunnel: [_ w427] -> _
      tunnel: w421 -> [_ _]
      frame False {
      }
      frame True {
        n221 = call "配置初始化.vi"() -> ("error out"=w427:errorcluster)  [unwired: 11 in]
      }
    }
  }
  n222 = flat-sequence {
    tunnel: w7 -> [_]
    frame #0 {
      (unwired) u32 0 ("等待时间（毫秒）")
      n223 = control-ref of="周期设置"() -> (w432:refnum<vi>)
      n224 = call "试剂余量后台任务.vi"() -> ()  [unwired: 12 in]
      n225 = call "New TimingControl.vi"("Reference"=w432) -> ("error out"=w430:errorcluster, "TimingControl out"=w431:refnum<class "TimingControl.lvclass">)  [unwired: 9 in]
      n226 = call "taskqueue ref.vi"() -> ("队列输出"=w433:refnum<queue>)  [unwired: 10 in, 1 out]
      n227 = while {
        tunnel: w433 -> [w452]
        shift-right: [w445] -> w429
        shift-left: w431 -> [w450]
        shift-right: [w444] -> w428
        shift-left: w430 -> [w449]
        stop <- FALSE stop-if-true
        n228 = global read "VAR总磷总氮全局变量.vi" "状态告警区"() -> (w453:T4)
        n229 = Wait (ms)(milliseconds to wait=u32 500 ("等待时间（毫秒）")) -> ()  [unwired: 1 out]
        n230 = global read "model config var.vi" "启动队列名称"() -> (w439:cluster{"String":string, "Value":u16}[])
        n231 = Unbundle By Name(w453) -> ("工作状态"=w451:u16, "系统时间"=w447:timestamp)
        n232 = for {
          tunnel: w439 -> [w464] mode=indexing
          tunnel: [w463] -> w438 mode=indexing
          n233 = Unbundle By Name(w464) -> ("String"=w463:string)
        }
        n234 = case shown="1, Default" w451 {
          tunnel: [FALSE TRUE] -> w446
          frame 0 {
          }
          frame 1, Default {
          }
        }
        n235 = property class="TimingControl"(reference=w450, error in=w449, "Properties:仪器时间"=w447, "Properties:仪器运行状态"=w446) -> (reference out=w445:refnum<class "TimingControl.lvclass">, error out=w444:errorcluster, "Properties:命令输出"=w448:cluster{"启动":bool, "控制命令":T12, "测量参数":T13})
        n236 = Array To Spreadsheet String(delimiter (Tab)="/" ("分隔符(Tab)"), array=w438, 3:"" ("格式字符串")) -> (spreadsheet string=w441:string)
        n237 = Unbundle By Name(w448) -> ("启动"=w435:bool, "控制命令"=w437:T12)
        n238 = Insert Into Array(array=w438, new element=w441) -> (w440:string[])  [unwired: 1 in]
        n239 = Bundle(w440) -> ()  [unwired: 1 in, 1 out]
        n240 = Bundle("控制命令"=w437, "") -> (w436:cluster{"控制命令":T12, string})  [unwired: 1 in]
        n241 = case shown="True" w435 {
          tunnel: w436 -> [_ w457]
          tunnel: w452 -> [_ w460]
          frame False {
          }
          frame True {
            n242 = Get Queue Status(queue=w460) -> (queue out=w458:refnum<queue>, # elements in queue=w459:i32)  [unwired: 2 in, 6 out]
            n243 = Equal To 0?(x=w459) -> (x = 0?=w456:bool)
            n244 = case shown="True" w456 {
              tunnel: w458 -> [_ w462]
              tunnel: w457 -> [_ w461]
              frame False {
              }
              frame True {
                n245 = Enqueue Element(queue=w462, element=w461) -> ()  [unwired: 2 in, 3 out]
              }
            }
          }
        }
      }
      n246 = call "task.vi"() -> ()  [unwired: 12 in]
      n247 = call "Close TimingControl.vi"("error in (no error)"=w428, "TimingControl in"=w429) -> ()  [unwired: 9 in, 1 out]
    }
  }
  n248 = while {
    tunnel: w7 -> [_]
    stop <- FALSE stop-if-true
    n249 = flat-sequence {
      frame #0 {
        n250 = global read "model config var.vi" "启动队列名称"() -> (w468:cluster{"String":string, "Value":u16}[])
        n251 = for {
          tunnel: w468 -> [w476] mode=indexing
          shift-right: [w475] -> w471
          shift-left: "" -> [w474]
          tunnel: [w473] -> w469 mode=indexing
          n252 = Unbundle By Name(w476) -> ("String"=w473:string)
          n253 = Concatenate Strings(w474, w473) -> (w475:string)
        }
        n254 = property on="单选按钮" class="RadioBtnsControl (strict)"() -> ("Controls[]"=w470:refnum<vi>[])  [unwired: 2 in, 2 out]
        n255 = global write "VAR总磷总氮全局变量.vi" "模块名称"(w471) -> ()
        n256 = for {
          tunnel: w470 -> [w484] mode=indexing
          tunnel: w469 -> [w483]
          n257 = property class="Ctl"(reference=w484) -> (reference out=w482:refnum<vi>, "Label.Text"=w478:string)  [unwired: 1 in, 1 out]
          n258 = case shown="\"COD\"" w478 {
            selector: w478 -> [w485 _]
            tunnel: [w485 "CODcr"] -> w477
            frame Default {
            }
            frame "COD" {
            }
          }
          n259 = Search 1D Array(1D array=w483, element=w477) -> (index of element=w481:i32)  [unwired: 1 in]
          n260 = Not Equal?(x=w481, y=-1) -> (x != y?=w479:bool)
          n261 = property class="Ctl"(reference=w482, "Visible"=w479) -> ()  [unwired: 1 in, 2 out]
        }
      }
      frame #1 {
        n262 = Wait (ms)(milliseconds to wait=u32 1000 ("等待时间（毫秒）")) -> ()  [unwired: 1 out]
      }
    }
  }
  n263 = call "时间延迟"("error in (no error)"=w6) -> ("error out"=w26:errorcluster)  [unwired: 10 in]
  n264 = vi-ref "斯坦道总氮.lvlib:校准设置页.vi"() -> (w15:refnum<vi>)
  n265 = vi-ref "斯坦道总氮.lvlib:参数设置页.vi"() -> (w19:refnum<vi>)
  n266 = property class="VI"(reference=w15, error in=w10) -> (reference out=w13:refnum<vi>, "Exec.State"=w14:T14)  [unwired: 1 out]
  n267 = property class="VI"(reference=w19, error in=w11) -> (reference out=w17:refnum<vi>, "Exec.State"=w18:T14)  [unwired: 1 out]
  n268 = while {
    tunnel: w26 -> [_]
    stop <- FALSE stop-if-true
    n269 = Wait (ms)(milliseconds to wait=u32 1000 ("等待时间（毫秒）")) -> ()  [unwired: 1 out]
    n270 = global read "VAR总磷总氮全局变量.vi" "状态告警区"() -> (w513:T4)
    n271 = global read "VAR总磷总氮全局变量.vi" "状态告警区"() -> (w514:T4)
    n272 = global read "VAR总磷总氮全局变量.vi" "状态告警区"() -> (w512:T4)
    n273 = global read "VAR总磷总氮全局变量.vi" "状态告警区"() -> (w510:T4)
    n274 = Unbundle By Name(w514) -> ("F0"=→"F0":sgl, "F1"=→"F1":sgl, "F2"=→"F2":sgl, "F3"=→"F3":sgl, "ADC"=→"ADC":sgl, "总磷控温温度1"=→"消解温度":sgl, "营养盐控温温度2"=→"注射器温度":sgl)
    n275 = Unbundle By Name(w513) -> ("日志代码"=w488:u16)
    "步骤" <- w488
    n276 = Unbundle By Name(w510) -> ("日志代码"=w509:u16)
    n277 = Unbundle By Name(w512) -> ("flowid"=w492:u16, "工作状态"=w505:u16, "id"=w506:u16)
    n278 = case shown="0" w505 {
      frame 0 {
        n279 = local write "数组"(string[] [] ("数组")) -> ()
      }
      frame 1, Default {
      }
    }
    n280 = feedback #4() -> (w511:u16)  [unwired: 1 in]
    n281 = feedback-in #4(w509) -> ()
    n282 = Not Equal To 0?(x=w505) -> (x != 0?=w490:bool)
    n283 = property on="总步数" class="DigNum (strict)"() -> ("Value"=w495:i32)  [unwired: 2 in, 2 out]
    n284 = Divide(x=w488, y=w495) -> (x/y=w494:dbl)
    n285 = Not Equal?(x=w509, y=w511) -> (x != y?=w508:bool)
    n286 = call <vilib>:"Boolean Crossing PtByPt.vi"("direction"=enum16{"either", "false-true", "true-false"}."either", "input"=w490) -> ("crossing"=w503:bool)  [unwired: 1 in]
    n287 = feedback-in #5(w488) -> ()
    n288 = feedback #5() -> (w516:u16)  [unwired: 1 in]
    n289 = Subtract(x=w488, y=1) -> (x-y=→"多列列表框":i32)
    n290 = case shown="True" w503 {
      tunnel: w506 -> [_ w539]
      tunnel: w492 -> [_ w527]
      tunnel: w490 -> [_ w525]
      frame False {
      }
      frame True {
        n291 = global read "VAR总磷总氮全局变量.vi" "最近一次工作状态"() -> (w526:u16)
        n292 = case shown="3" w526 {
          selector: w526 -> [w545 _ _ _ _ _ _ _ _ _ _ _]
          tunnel: [w544 "【水样测试】" ("字符串") w548 "【零点核查】" ("字符串") "【跨度核查】" ("字符串") "【空白测试】" ("字符串") "【平行样测试】" ("字符串") "【加标回收】" ("字符串") "【空白校准】" ("字符串") "【标样校准】" ("字符串") "【单步调试】" ("字符串") "【简易流程】" ("字符串")] -> w520
          tunnel: w527 -> [_ _ w547 _ _ _ _ _ _ _ _ _]
          frame 0, Default {
            n293 = Number To Decimal String(number=w545) -> (decimal integer string=w544:string)  [unwired: 1 in]
          }
          frame 1 {
          }
          frame 2 {
            n294 = case shown="0, Default" w547 {
              tunnel: ["【标样核查】" ("字符串") "【快捷测试】" ("字符串")] -> w548
              frame 0, Default {
              }
              frame 5 {
              }
            }
          }
          frame 3 {
          }
          frame 4 {
          }
          frame 5 {
          }
          frame 6 {
          }
          frame 7 {
          }
          frame 8 {
          }
          frame 9 {
          }
          frame 254 {
          }
          frame 255 {
          }
        }
        n295 = global read "VAR总磷总氮全局变量.vi" "状态告警区"() -> (w537:T4)
        n296 = Concatenate Strings("<<" ("字符串"), w520, "启动" ("字符串")) -> (w519:string)
        n297 = Unbundle By Name(w537) -> ("F0"=w536:sgl, "F1"=w535:sgl, "F2"=w534:sgl, "F3"=w533:sgl, "id"=w532:u16, "flowid"=w531:u16, "量程"=w530:u16)
        n298 = Concatenate Strings(w520, "停止>>" ("字符串")) -> (w523:string)
        n299 = Format Into String(format string="F0=%#f,F1=%#f,F2=%#f,F3=%#f,Flow=%d-%-d-%-d" ("格式字符串"), w536, w535, w534, w533, w532, w531, w530) -> (resulting string=w528:string)  [unwired: 2 in, 1 out]
        n300 = Select(t=w519, s=w525, f=w523) -> (s? t:f=w524:string)
        n301 = call "id参数转换.vi"("id"=w539) -> ("table输出"=w538:string)  [unwired: 9 in, 1 out]
        n302 = Get Date/Time In Seconds() -> (seconds since 1Jan1904=w542:timestamp)
        n303 = Bundle By Name(cluster=T15 {"时间标识"=timestamp(0 s since 1904-01-01), "设备"="", "日志信息"="", "流程参数"=""} ("data in"), "时间标识"=w542, "设备"=w538, "日志信息"=w524, "流程参数"=w528) -> (w541:T15)
        n304 = call "总磷总氮操作日志.vi"("data in"=w541) -> ()  [unwired: 10 in, 1 out]
      }
    }
    n305 = case shown="True" w508 {
      frame False {
      }
      frame True {
        n306 = property on="多列列表框" class="MCListbox (strict)"() -> ("ItemNames"=w565:string[][], "Value"=w561:i32)  [unwired: 2 in, 2 out]
        n307 = Index Array(array=w565, index (row)=w561) -> (element=w564:string[])  [unwired: 1 in]
        n308 = Index Array(array=w564) -> (element=w563:string)  [unwired: 1 in]
        n309 = call "过滤筛选流程.vi"("字符串"=w563) -> ("匹配后偏移量"=w562:i32)  [unwired: 10 in]
        n310 = case shown="Default" w562 {
          tunnel: w563 -> [w567 _]
          tunnel: w561 -> [w566 _]
          frame Default {
            n311 = case shown="\"读数\"" w567 {
              selector: w567 -> [w573 w580]
              tunnel: [w573 w580] -> w569
              tunnel: [string[] [] ("数组") w575] -> w568
              tunnel: w566 -> [_ w579]
              frame "读数" {
              }
              frame Default {
                n312 = Equal?(x=w579, y=1) -> (x = y?=w577:bool)
                n313 = Select(t=string[] [], s=w577, f="数组") -> (s? t:f=w575:string[])
              }
            }
            n314 = for {
              N: 1 -> [_]
              tunnel: w569 -> [w582]
              shift-right: [w581] -> w570
              shift-left: w568 -> [w583]
              n315 = Search 1D Array(1D array=w583, element=w582) -> (index of element=w586:i32)  [unwired: 1 in]
              n316 = Format Into String(format string="%s" ("格式字符串"), w582) -> (resulting string=w587:string)  [unwired: 2 in, 1 out]
              n317 = Equal?(x=w586, y=-1) -> (x = y?=w584:bool)
              n318 = case shown="True" w584 {
                tunnel: w587 -> [_ w597]
                tunnel: w583 -> [w589 w601]
                tunnel: w582 -> [_ w600]
                tunnel: [w589 w599] -> w581
                frame False {
                }
                frame True {
                  n319 = Insert Into Array(array=w601, new element=w600) -> (w599:string[])  [unwired: 1 in]
                  n320 = global read "VAR总磷总氮全局变量.vi" "状态告警区"() -> (w596:T4)
                  n321 = Unbundle By Name(w596) -> ("工作状态"=w595:u16, "flowid"=w590:u16)
                  n322 = case shown="2" w595 {
                    selector: w595 -> [w616 _ _ _ _ _ _ _ _ _ _ _]
                    tunnel: [w615 "【水样测试】" ("字符串") w619 "【零点核查】" ("字符串") "【跨度核查】" ("字符串") "【空白测试】" ("字符串") "【平行样测试】" ("字符串") "【加标回收】" ("字符串") "【空白校准】" ("字符串") "【标样校准】" ("字符串") "【单步调试】" ("字符串") w630] -> w593
                    tunnel: w590 -> [_ _ w618 _ _ _ _ _ _ _ _ _]
                    frame 0, Default {
                      n323 = Number To Decimal String(number=w616) -> (decimal integer string=w615:string)  [unwired: 1 in]
                    }
                    frame 1 {
                    }
                    frame 2 {
                      n324 = case shown="5" w618 {
                        tunnel: ["【标样核查】" ("字符串") "【快捷测试】" ("字符串")] -> w619
                        frame Default {
                        }
                        frame 5 {
                        }
                      }
                    }
                    frame 3 {
                    }
                    frame 4 {
                    }
                    frame 5 {
                    }
                    frame 6 {
                    }
                    frame 7 {
                    }
                    frame 8 {
                    }
                    frame 9 {
                    }
                    frame 254 {
                    }
                    frame 255 {
                      n325 = local read "简易步骤名称"() -> (w632:string)
                      n326 = Format Into String(format string="(%s)" ("格式字符串"), initial string="【简易流程】" ("工作状态"), w632) -> (resulting string=w630:string)  [unwired: 1 in, 1 out]
                    }
                  }
                  n327 = global read "VAR总磷总氮全局变量.vi" "状态告警区"() -> (w614:T4)
                  n328 = global read "VAR总磷总氮全局变量.vi" "状态告警区"() -> (w611:T4)
                  n329 = Unbundle By Name(w611) -> ("F0"=w608:sgl, "F1"=w607:sgl, "F2"=w606:sgl, "F3"=w605:sgl, "id"=w604:u16, "flowid"=w603:u16, "量程"=w602:u16)
                  n330 = Unbundle By Name(w614) -> ("id"=w592:u16)
                  n331 = call "id参数转换.vi"("id"=w592) -> ("table输出"=w591:string)  [unwired: 9 in, 1 out]
                  n332 = Concatenate Strings(w593, w597) -> (w594:string)
                  n333 = Format Into String(format string="F0=%#f,F1=%#f,F2=%#f,F3=%#f,Flow=%d-%-d-%-d" ("格式字符串"), w608, w607, w606, w605, w604, w603, w602) -> (resulting string=w609:string)  [unwired: 2 in, 1 out]
                  n334 = Get Date/Time In Seconds() -> (seconds since 1Jan1904=w612:timestamp)
                  n335 = Bundle By Name(cluster=T15 {"时间标识"=timestamp(0 s since 1904-01-01), "设备"="", "日志信息"="", "流程参数"=""} ("data in"), "时间标识"=w612, "设备"=w591, "日志信息"=w594, "流程参数"=w609) -> (w613:T15)
                  n336 = call "总磷总氮操作日志.vi"("data in"=w613) -> ()  [unwired: 10 in, 1 out]
                }
              }
            }
            n337 = local write "数组"(w570) -> ()
          }
          frame -1 {
          }
        }
      }
    }
    n338 = Not Equal?(x=w488, y=w516) -> (x != y?=w515:bool)
    n339 = Multiply(x=w494, y=100.0) -> (x*y=w491:dbl)
    "滑动杆" <- w491
    n340 = case shown="True" w515 {
      tunnel: w488 -> [_ w636]
      frame False {
      }
      frame True {
        n341 = Subtract(x=w636, y=1) -> (x-y=w634:i32)
        n342 = Subtract(x=w634, y=5) -> (x-y=w638:i32)
        n343 = Greater Or Equal To 0?(x=w638) -> (x >= 0?=w637:bool)
        n344 = property on="多列列表框" class="MCListbox (strict)"() -> (error out=w642:errorcluster, "TopLeft"=w643:T16)  [unwired: 2 in, 1 out]
        n345 = Select(t=w638, s=w637, f=0) -> (s? t:f=w639:i32)
        n346 = Bundle By Name(cluster=w643, "Row"=w639) -> (w644:T16)
        n347 = property on="多列列表框" class="MCListbox (strict)"(error in=w642, "TopLeft"=w644) -> ()  [unwired: 1 in, 2 out]
      }
    }
    n348 = global write "VAR总磷总氮全局变量.vi" "测试进度"(w491) -> ()
  }
  n349 = case shown="\"Idle\"" w14 {
    tunnel: w13 -> [w645 w649]
    tunnel: [w645 w646] -> w12
    frame "Bad", Default {
    }
    frame "Idle" {
      n350 = invoke class="VI" method="Run VI"(reference=w649, "Wait until done"=FALSE ("结束前等待"), "Auto Dispose Ref"=TRUE ("自动销毁引用")) -> (reference out=w646:refnum<vi>)  [unwired: 2 in, 4 out]
    }
  }
  n351 = case shown="\"Idle\"" w18 {
    tunnel: w17 -> [w650 w654]
    tunnel: [w650 w651] -> w16
    frame "Bad", Default {
    }
    frame "Idle" {
      n352 = invoke class="VI" method="Run VI"(reference=w654, "Wait until done"=FALSE ("结束前等待"), "Auto Dispose Ref"=TRUE ("自动销毁引用")) -> (reference out=w651:refnum<vi>)  [unwired: 2 in, 4 out]
    }
  }
  n353 = Obtain Notifier(name (unnamed)=w20, notification data type=FALSE) -> (notifier out=w21:refnum<notifier>)  [unwired: 2 in, 2 out]
  n354 = Obtain Queue(name (unnamed)=w20, element data type=cluster{"命令":string, "data":variant} {"命令"="", "data"=variant}) -> (queue out=w23:refnum<queue>)  [unwired: 3 in, 2 out]
  n355 = while {
    tunnel: w23 -> [w658]
    tunnel: w21 -> [w657]
    tunnel: w16 -> [w656]
    tunnel: w12 -> [w655]
    stop <- FALSE stop-if-true
    n356 = event shown="[8] \"手动启动\": Value Change" {
      selector: _ -> [_ _ _ _ _ _ _ _ _ _ _ _ _ _]
      dyn-events: _ -> [_ _ _ _ _ _ _ _ _ _ _ _ _ _]
      timeout: _ -> [_ _ _ _ _ _ _ _ _ _ _ _ _ _]
      tunnel: w658 -> [_ _ _ _ _ _ _ _ w672 _ w679 _ _ _]
      tunnel: w657 -> [_ _ _ _ _ _ _ _ _ _ w678 _ _ _]
      tunnel: w656 -> [_ _ _ _ _ _ _ _ _ _ _ w699 _ _]
      tunnel: w655 -> [_ _ _ _ _ _ _ _ _ _ _ _ w705 _]
      event Timeout {
        n357 = event-data() -> ()  [unwired: 1 in, 3 out]
      }
      event "流程操作": Value Change {
        n358 = event-data() -> ()  [unwired: 1 in, 6 out]
        n359 = global read "总磷总氮断电保存全局变量.vi" "简易流程路径"() -> (w660:path)
        n360 = global read "总磷总氮断电保存全局变量.vi" "流程路径"() -> (w661:path)
        n361 = call "流程批量写入.vi"("简易流程路径"=w660, "添加的路径"=w661) -> ()  [unwired: 10 in]
      }
      event "温度曲线": Value Change {
        n362 = event-data() -> ()  [unwired: 1 in, 6 out]
        n363 = call "温度曲线显示.vi"() -> ()  [unwired: 12 in]
      }
      event "试剂余量": Value Change {
        n364 = event-data() -> ()  [unwired: 1 in, 6 out]
        n365 = call "试剂余量显示UI.vi"() -> ()  [unwired: 12 in]
      }
      event "灯值调整": Value Change {
        n366 = event-data() -> ()  [unwired: 1 in, 6 out]
        n367 = call "灯值调整对话框.vi"() -> ()  [unwired: 12 in]
      }
      event "布尔": Value Change {
        n368 = event-data() -> ("NewVal"=w662:bool)  [unwired: 1 in, 5 out]
        n369 = case shown="False" w662 {
          frame False {
            n370 = global write "VAR总磷总氮全局变量.vi" "权限等级"(enum16{"一级权限", "二级权限", "三级权限", "超级权限"}."一级权限" ("权限等级")) -> ()
          }
          frame True {
            n371 = global read "VAR总磷总氮全局变量.vi" "权限密码"() -> (w666:u32[])
            n372 = global read "VAR总磷总氮全局变量.vi" "权限等级"() -> (w664:enum16{"一级权限", "二级权限", "三级权限", "超级权限"})
            n373 = call "密码权限设置.vi"("权限输入"=w664, "权限密码"=w666) -> ("权限输出"=w665:enum16{"一级权限", "二级权限", "三级权限", "超级权限"})  [unwired: 9 in]
            n374 = global write "VAR总磷总氮全局变量.vi" "权限等级"(w665) -> ()
          }
        }
      }
      event "权限等级": Mouse Down {
        n375 = event-data() -> ()  [unwired: 1 in, 8 out]
        n376 = global read "VAR总磷总氮全局变量.vi" "权限密码"() -> (w669:u32[])
        n377 = global read "VAR总磷总氮全局变量.vi" "权限等级"() -> (w667:enum16{"一级权限", "二级权限", "三级权限", "超级权限"})
        n378 = call "密码权限设置.vi"("权限输入"=w667, "权限密码"=w669) -> ("权限输出"=w668:enum16{"一级权限", "二级权限", "三级权限", "超级权限"})  [unwired: 9 in]
        n379 = global write "VAR总磷总氮全局变量.vi" "权限等级"(w668) -> ()
      }
      event "外设固件": Value Change {
        n380 = event-data() -> ()  [unwired: 1 in, 6 out]
        n381 = call "流程固件设置对话框.vi"() -> ()  [unwired: 12 in]
      }
      event "手动启动": Value Change {
        n382 = event-data() -> ()  [unwired: 1 in, 6 out]
        n383 = call "总磷总氮启动参数对话框.vi"() -> ("确认"=w670:bool, "元素"=w671:cluster{"命令":string, "data":variant})  [unwired: 10 in]
        n384 = case shown="True" w670 {
          tunnel: w672 -> [_ w675]
          tunnel: w671 -> [_ w674]
          frame False {
          }
          frame True {
            n385 = Flush Queue(queue=w675) -> (queue out=w673:refnum<queue>)  [unwired: 1 in, 2 out]
            n386 = Enqueue Element(queue=w673, element=w674) -> ()  [unwired: 2 in, 3 out]
          }
        }
      }
      event "调试": Value Change {
        n387 = event-data() -> ()  [unwired: 1 in, 6 out]
        n388 = call "简易流程调试界面.vi"() -> ()  [unwired: 12 in]
      }
      event "停止": Value Change {
        n389 = event-data() -> ()  [unwired: 1 in, 6 out]
        n390 = Two Button Dialog(message="确认停止？" ("消息")) -> (T button?=w676:bool)  [unwired: 2 in]
        n391 = case shown="True" w676 {
          tunnel: w679 -> [_ w695]
          tunnel: w678 -> [_ w694]
          frame False {
          }
          frame True {
            n392 = Send Notification(notification=TRUE ("通知"), notifier=w694) -> ()  [unwired: 1 in, 2 out]
            n393 = global read "VAR总磷总氮全局变量.vi" "状态告警区"() -> (w689:T4)
            n394 = global read "VAR总磷总氮全局变量.vi" "状态告警区"() -> (w681:T4)
            n395 = Unbundle By Name(w689) -> ("id"=w688:u16)
            n396 = Unbundle By Name(w681) -> ("id"=w680:u16)
            n397 = Bundle By Name(cluster=T18 {"站号"=1, "量程切换"=enum."AUTO", "控制命令"=enum."停止测试", "模式设置"=enum."待机", "测量间隔"=0} ("参数"), "站号"=w688) -> (w690:T18)
            n398 = call "id参数转换.vi"("id"=w680) -> ("table输出"=w682:string)  [unwired: 9 in, 1 out]
            n399 = call "总磷总氮启动命令.vi"("参数"=w690) -> ("启动命令"=w691:cluster{"命令":string, "data":variant})  [unwired: 10 in]
            n400 = Get Date/Time In Seconds() -> (seconds since 1Jan1904=w685:timestamp)
            n401 = Bundle By Name(cluster=T17 {"时间"=timestamp(0 s since 1904-01-01), "参数"="", "日志信息"="", "流程参数"=""} ("data in"), "时间"=w685, "参数"=w682, "日志信息"="手动停止") -> (w686:T17)
            n402 = Enqueue Element(queue=w695, element=w691) -> (error out=w683:errorcluster)  [unwired: 2 in, 2 out]
            n403 = call "总磷总氮操作日志.vi"("错误输入（无错误）"=w683, "data in"=w686) -> ()  [unwired: 9 in, 1 out]
          }
        }
      }
      event "参数设置", "参数查询": Value Change {
        n404 = event-data() -> ()  [unwired: 1 in, 6 out]
        n405 = invoke on="子面板" class="SubPnl" method="Remove VI"() -> (error out=w700:errorcluster)  [unwired: 3 in, 2 out]
        n406 = property on="仪器校准" class="Bool"("Visible"=TRUE ("可见")) -> ()  [unwired: 2 in, 2 out]
        n407 = property on="参数查询" class="Bool"("Visible"=FALSE ("可见")) -> ()  [unwired: 2 in, 2 out]
        n408 = property on="窗格" class="Pane"("Origin"=T6 {"Horizontal"=0, "Vertical"=640} ("原点")) -> ()  [unwired: 2 in, 2 out]
        n409 = invoke on="子面板" class="SubPnl" method="Insert VI"(error in=w700, "VI Ref"=w699) -> ()  [unwired: 2 in, 4 out]
        n410 = global write "VAR总磷总氮全局变量.vi" "页面"(enum16{"主页", "参数页", "校准页"}."参数页" ("页面")) -> ()
      }
      event "仪器校准": Value Change {
        n411 = event-data() -> ()  [unwired: 1 in, 6 out]
        n412 = invoke on="子面板" class="SubPnl" method="Remove VI"() -> (error out=w706:errorcluster)  [unwired: 3 in, 2 out]
        n413 = property on="仪器校准" class="Bool"("Visible"=FALSE ("可见")) -> ()  [unwired: 2 in, 2 out]
        n414 = property on="参数查询" class="Bool"("Visible"=TRUE ("可见")) -> ()  [unwired: 2 in, 2 out]
        n415 = global write "VAR总磷总氮全局变量.vi" "页面"(enum16{"主页", "参数页", "校准页"}."校准页" ("页面")) -> ()
        n416 = invoke on="子面板" class="SubPnl" method="Insert VI"(error in=w706, "VI Ref"=w705) -> ()  [unwired: 2 in, 4 out]
      }
      event "返回": Value Change {
        n417 = event-data() -> ()  [unwired: 1 in, 6 out]
        n418 = global write "VAR总磷总氮全局变量.vi" "页面"(enum16{"主页", "参数页", "校准页"}."主页" ("页面")) -> ()
        n419 = property on="窗格" class="Pane"("Origin"=T6 {"Horizontal"=0, "Vertical"=0} ("原点")) -> ()  [unwired: 2 in, 2 out]
      }
    }
  }
  n420 = while {
    tunnel: w23 -> [w720]
    stop <- FALSE stop-if-true
    n421 = Wait (ms)(milliseconds to wait=u32 1000 ("等待时间（毫秒）")) -> ()  [unwired: 1 out]
    n422 = global read "总磷总氮断电保存全局变量.vi" "MB通信方式选择"() -> (w718:enum16{"串口", "TCP"})
    n423 = global read "VAR总磷总氮全局变量.vi" "升级固件关闭心跳包"() -> (w712:bool)
    n424 = global read "VAR总磷总氮全局变量.vi" "MB session in"() -> (w716:refnum<class "MB_Master.lvclass">)
    n425 = case shown="\"串口\", Default" w718 {
      tunnel: [w723 w724] -> w717
      frame "串口", Default {
        n426 = global read "总磷总氮断电保存全局变量.vi" "VISA Resource"() -> (w723:refnum<visa-resource-name>)
      }
      frame "TCP" {
        n427 = global read "总磷总氮断电保存全局变量.vi" "IP"() -> (w724:string)
      }
    }
    "字符串 2" <- w717
    n428 = property class="MB_Master"(reference=w716) -> ("Properties:Session Valid"=w714:bool)  [unwired: 1 in, 2 out]
    n429 = Not(x=w712) -> (.not. x?=w711:bool)
    n430 = Get Queue Status(queue=w720) -> (queue out=w719:refnum<queue>, # elements in queue=w715:i32)  [unwired: 2 in, 6 out]
    n431 = Equal To 0?(x=w715) -> (x = 0?=w709:bool)
    n432 = Compound Arithmetic op=AND ("复合运算")(w714, w711) -> (w713:bool)
    n433 = global write "VAR总磷总氮全局变量.vi" "心跳包打开状态"(w713) -> ()
    n434 = And(x=w709, y=w713) -> (x .and. y?=w710:bool)
    n435 = case shown="True" w710 {
      tunnel: w719 -> [_ w743]
      frame False {
      }
      frame True {
        n436 = global read "VAR总磷总氮全局变量.vi" "MB session in"() -> (w731:refnum<class "MB_Master.lvclass">)
        n437 = property class="MB_Master"(reference=w731) -> ("Properties:Session Valid"=w729:bool)  [unwired: 1 in, 2 out]
        n438 = global read "VAR总磷总氮全局变量.vi" "通讯状态"() -> (w732:bool)
        n439 = case shown="True" w729 {
          tunnel: [_ w745] -> w728
          frame False {
          }
          frame True {
            n440 = global read "VAR总磷总氮全局变量.vi" "MB session in"() -> (w744:refnum<class "MB_Master.lvclass">)
            n441 = call "版本号读取.vi"("MB session in"=w744) -> ("error out"=w745:errorcluster, "固件版本号"=w746:string)  [unwired: 8 in, 1 out]
            "固件版本号" <- w746
            n442 = global write "VAR总磷总氮全局变量.vi" "固件版本号"(w746) -> ()
          }
        }
        n443 = And(x=w729, y=w732) -> (x .and. y?=w730:bool)
        n444 = case shown="True" w730 {
          tunnel: [_ w747] -> w727
          tunnel: w728 -> [_ w748]
          frame False {
          }
          frame True {
            n445 = global read "VAR总磷总氮全局变量.vi" "MB session in"() -> (w750:refnum<class "MB_Master.lvclass">)
            n446 = call "序列号读取.vi"("Error in"=w748, "MB session in"=w750) -> ("error out"=w747:errorcluster, "序列号"=w749:string)  [unwired: 7 in, 1 out]
            n447 = global write "VAR总磷总氮全局变量.vi" "序列号"(w749) -> ()
          }
        }
        n448 = global read "model config var.vi" "启动队列名称"() -> (w734:cluster{"String":string, "Value":u16}[])
        n449 = for {
          tunnel: [w761] -> w735 mode=indexing
          tunnel: w734 -> [w762] mode=indexing
          tunnel: w727 -> [_]
          n450 = Unbundle By Name(w762) -> ("Value"=w761:u16)
        }
        n451 = for {
          shift-right: [w751] -> w737
          shift-left: w743 -> [w757]
          tunnel: w735 -> [w752] mode=indexing
          n452 = Bundle By Name(cluster=cluster{"命令":string, "data":variant} {"命令"="", "data"=variant} ("元素"), "命令"="读状态告警区", "data"=w752) -> (w759:cluster{"命令":string, "data":variant})
          n453 = Bundle By Name(cluster=cluster{"命令":string, "data":variant} {"命令"="", "data"=variant} ("元素"), "命令"="读测量数据区", "data"=w752) -> (w754:cluster{"命令":string, "data":variant})
          n454 = Enqueue Element(queue=w757, element=w759) -> (queue out=w753:refnum<queue>)  [unwired: 2 in, 2 out]
          n455 = Enqueue Element At Opposite End(queue=w753, element=w754) -> (queue out=w751:refnum<queue>)  [unwired: 2 in, 2 out]
        }
        n456 = global read "VAR总磷总氮全局变量.vi" "状态告警区"() -> (w736:T4)
        n457 = Unbundle By Name(w736) -> ("系统时间"=w725:timestamp)
        n458 = Get Date/Time In Seconds() -> (seconds since 1Jan1904=w742:timestamp)
        n459 = Subtract(x=w742, y=w725) -> (x-y=w741:dbl)
        n460 = Absolute Value(x=w741) -> (abs(x)=w740:dbl)
        n461 = global read "VAR总磷总氮全局变量.vi" "通讯状态"() -> (w726:bool)
        n462 = Greater Or Equal?(x=w740, y=30.0) -> (x >= y?=w738:bool)
        n463 = Compound Arithmetic op=AND ("复合运算")(w738, w726) -> (w733:bool)
        n464 = case shown="True" w733 {
          tunnel: w737 -> [_ w764]
          frame False {
          }
          frame True {
            n465 = call "总磷总氮启动命令.vi"("参数"=T18 {"站号"=3, "量程切换"=enum."AUTO", "控制命令"=enum."校时", "模式设置"=enum."待机", "测量间隔"=0}) -> ("启动命令"=w763:cluster{"命令":string, "data":variant})  [unwired: 10 in]
            n466 = Enqueue Element(queue=w764, element=w763) -> ()  [unwired: 2 in, 3 out]
          }
        }
      }
    }
  }
